vi "detectie_stopstreep_al_dan_niet (SubVI).vi"(10 "OK Button":bool, 11 "ingegeven waardes reflectiesensor":dbl[](array[numeric])) -> (2 "Boolean":bool)   [LabVIEW 2019]
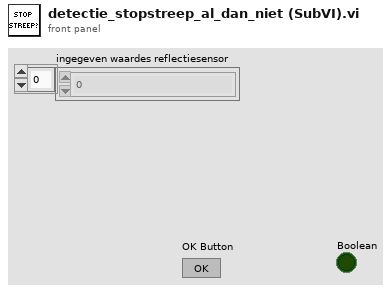
[diagram p1: front panel]
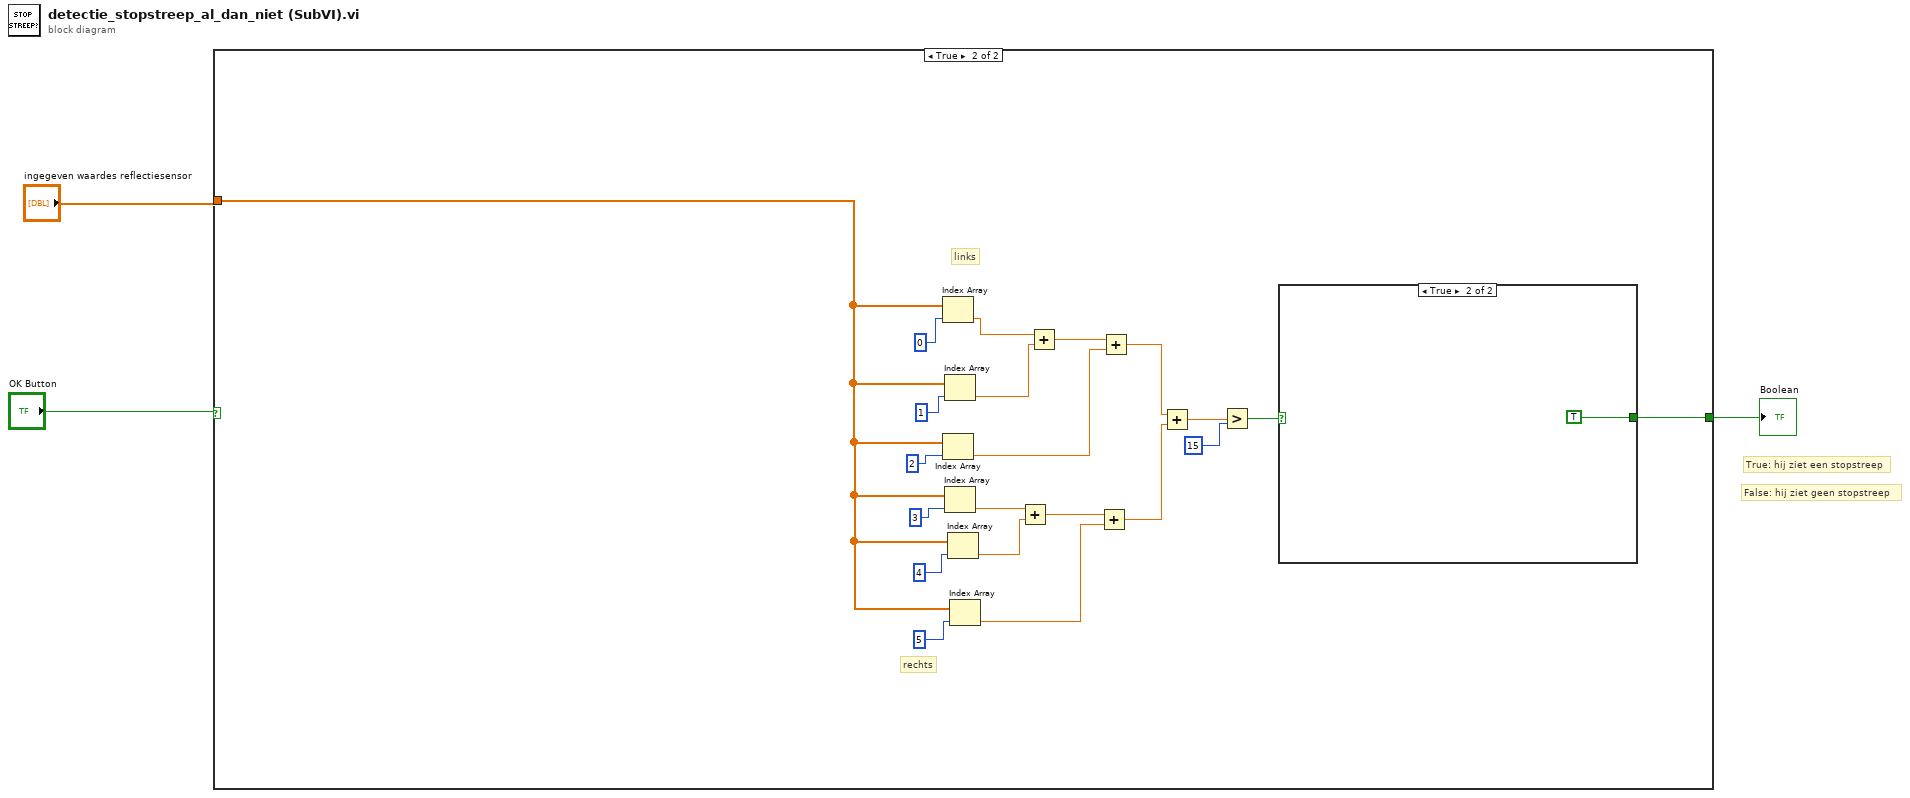
[diagram p0: block diagram]
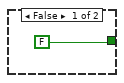
[diagram p2: hidden frame]
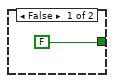
[diagram p3: hidden frame]
diagram:
  # "False: hij ziet geen stopstreep"
  # "True: hij ziet een stopstreep"
  n1 = case shown="True" "OK Button" {
    tunnel: [FALSE w6] -> w3
    tunnel: "ingegeven waardes reflectiesensor" -> [_ w5]
    frame False {
    }
    frame True {
      # "links"
      # "rechts"
      n2 = Index Array(array=w5, index=0) -> (element=w13:dbl)
      n3 = Index Array(array=w5, index=2) -> (element=w16:dbl)
      n4 = Index Array(array=w5, index=1) -> (element=w14:dbl)
      n5 = Index Array(array=w5, index=3) -> (element=w17:dbl)
      n6 = Index Array(array=w5, index=4) -> (element=w18:dbl)
      n7 = Index Array(array=w5, index=5) -> (element=w19:dbl)
      n8 = Add(x=w17, y=w18) -> (x+y=w20:dbl)
      n9 = Add(x=w13, y=w14) -> (x+y=w15:dbl)
      n10 = Add(x=w20, y=w19) -> (x+y=w22:dbl)
      n11 = Add(x=w15, y=w16) -> (x+y=w21:dbl)
      n12 = Add(x=w21, y=w22) -> (x+y=w23:dbl)
      n13 = Greater?(x=w23, y=15) -> (0:w25:bool)
      n14 = case shown="True" w25 {
        tunnel: [FALSE TRUE] -> w6
        frame False {
        }
        frame True {
        }
      }
    }
  }
  "Boolean" <- w3
